vi "OnDataChange.vi"(0 "DemoCameraController in":refnum<class "DemoCameraController.lvclass">, 1 "DataExchange":T1, 3 "error in (no error)":errorcluster) -> (7 "DemoCameraController out":refnum<class "DemoCameraController.lvclass">, 10 "error out":errorcluster)   [LabVIEW 2020, in "DemoCameraController.lvlib" / "DemoCameraController.lvclass"]
uses:
  DemoCameraController.lvclass
  Model/Hardware Abstraction Layer/Component/Device/Device/DataExchange.ctl
  Interface/DataListener/DataListener.lvclass
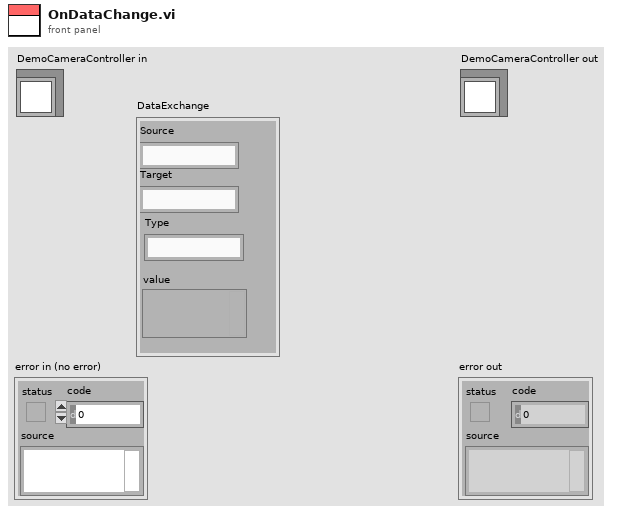
[diagram p1: front panel]
types:
  T1 = typedef "DataListener.lvclass/DataExchange.ctl" = cluster{"Source":string, "Target":string, "Type":string, "value":variant}
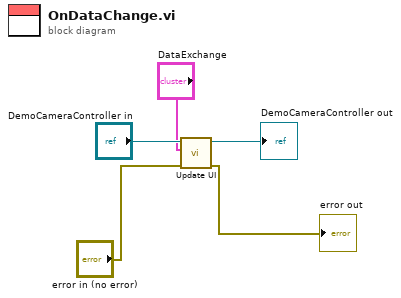
[diagram p0: block diagram]
diagram:
  n1 = call-dynamic "Update UI.vi"("error in (no error)"="error in (no error)", "DataExchange"="DataExchange", "Controller Template in"="DemoCameraController in") -> ("error out"=→"error out":errorcluster, "Controller Template out"=→"DemoCameraController out":refnum<class "DemoCameraController.lvclass">)  [unwired: 7 in]
